vi "CameraInterpreter.vi"() -> (1 "Overhead Image":T1(plugin-control), 2 "Boat Orientation":T2 scale=0.0..6.283, 3 "Boat Position":T3)   [LabVIEW 2011]
uses:
  2-RIO/2 Typedefs/Boat Position.ctl
  2-RIO/2 Typedefs/Boat Orientation.ctl
  <vilib>/vision/Image Controls.llb/IMAQ Image.ctl
panel:
  # "PLACEHOLDER VI\nPLACEHOLDER VI\nPLACEHOLDER VI"
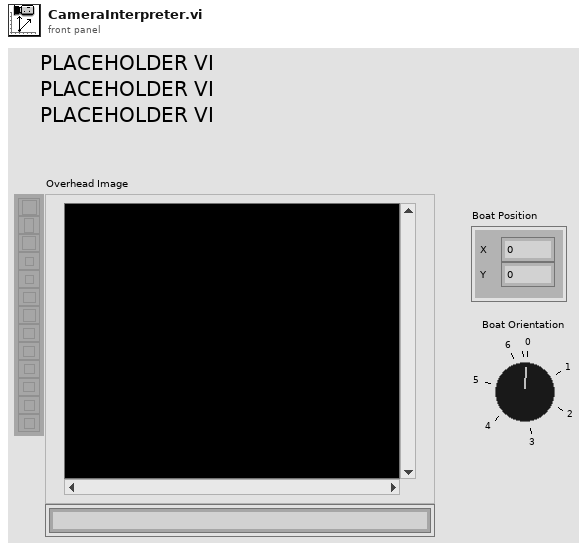
[diagram p1: front panel]
types:
  T1 = typedef "IMAQ Image.ctl" = refnum<image>
  T2 = typedef "Boat Orientation.ctl" = dbl
  T3 = typedef "Boat Position.ctl" = cluster{"X":dbl, "Y":dbl}
  T4 = cluster{"number: 0 to 1":dbl, "number: 0 to 1":dbl}
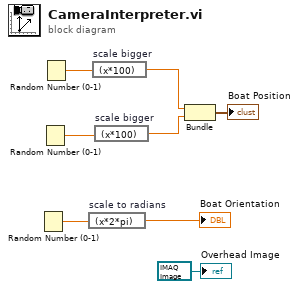
[diagram p0: block diagram]
diagram:
  n1 = Random Number (0-1)() -> (number: 0 to 1=w7:dbl)
  n2 = Random Number (0-1)() -> (number: 0 to 1=w5:dbl)
  n3 = Random Number (0-1)() -> (number: 0 to 1=w6:dbl)
  n4 = expression code="(x*2*pi)" "scale to radians"(w7) -> (→"Boat Orientation":dbl)
  n5 = expression code="(x*100)" "scale bigger"(w6) -> (w3:dbl)
  n6 = expression code="(x*100)" "scale bigger"(w5) -> (w2:dbl)
  n7 = Bundle("number: 0 to 1"=w3, "number: 0 to 1"=w2) -> (→"Boat Position":T4)  [unwired: 1 in]
  "Overhead Image" <- T1 refnum ("Image")
